vi "Main VI.vi"() -> ()   [LabVIEW 2015]
uses:
  Control 2.ctl
  <vilib>/MakerHub/LINX/Public/Peripherals/Digital/Digital Write 1 Chan.vi
  <vilib>/MakerHub/LINX/Public/Peripherals/Digital/Digital Write N Chans.vi
  <vilib>/MakerHub/LINX/Private/Local IO/LinxDigitalWrite.vi
  <vilib>/MakerHub/LINX/Public/Utilities/Check Channel.vi
  <vilib>/MakerHub/LINX/Public/Utilities/Open Serial.vi
  <vilib>/MakerHub/LINX/Private/Utilties/Generate Error.vi
  <vilib>/MakerHub/LINX/LMH-LINX.lvlib
panel:
  in  "Stop Button":bool caption="Blank Button"
  in  "Blank Button":bool
  out "7":bool
  out "6":bool
  out "5":bool
  out "4":bool
  out "3":bool
  out "2":bool
  in  "Select Pattern":T1(ring)=enum."All Blink"
  out "Error Details":errorcluster
  out "Device Name":string
  in  "Serial Port":refnum<visa-resource-name>="COM4"
  # "ARDUINO LED PATTERN PROGRAM v1.0"
  # "LED Pin Configuration"
  # "Pattern Selection"
  # "Board Settings"
  # "Error Details"
  # "Programmed by Aswin Sarang & Tarun Goyal\nwww.aswinsarang.com\nmail@aswinsarang.com"
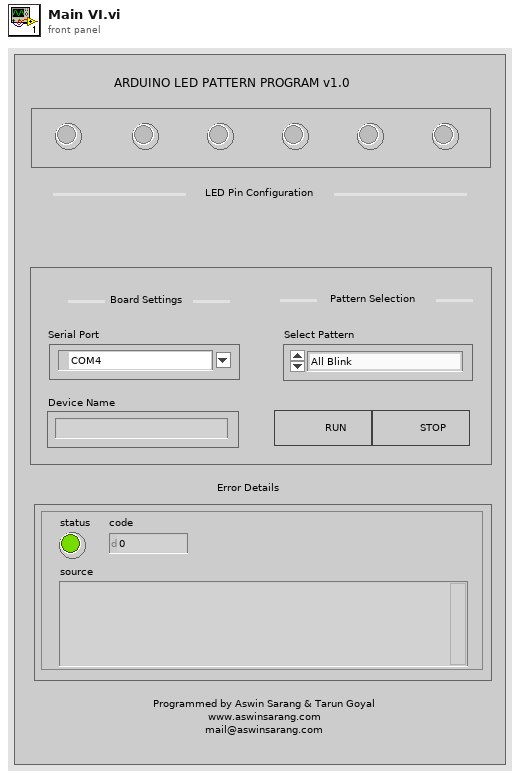
[diagram p1: front panel]
types:
  T1 = enum16{"Open & Close", "Odd & Even", "All Blink", "Running"}
  T2 = typedef "LMH-LINX.lvlib/LINX Ref.ctl" = cluster{"IO":T3, "Interface":T4, "LINX Device Config":T5}
  T3 = typedef "LMH-LINX.lvlib/Platform.ctl" = enum16{"Remote", "Local"}
  T4 = typedef "LMH-LINX.lvlib/Interface.ctl" = enum16{"Serial", "TCP"}
  T5 = typedef "LMH-LINX.lvlib/Device.lvlib/LINX Device Config.ctl" = cluster{"Interface":T4, "COM Port":refnum<visa-resource-name>, "TCP Configuration":T6, "Device Family":u8, "Device ID":u8, "Device Name":string, "TCP Ref":refnum<k5>, "Channels":T7}
  T6 = typedef "LMH-LINX.lvlib/Device.lvlib/TCP Config.ctl" = cluster{"IP Address":string, "Port":u16}
  T7 = typedef "LMH-LINX.lvlib/Channels.ctl" = cluster{"DI":u8[], "DO":u8[], "AI":u8[], "AO":u8[], "PWM":u8[], "QE":u8[], "UART":u8[], "I2C 2":u8[], "SPI":u8[], "CAN":u8[], "Servo":u8[], "AI Ref (V)":dbl, "AI Resolution (Bits)":u8, "AO Ref (V)":dbl, "AO Resolution (Bits)":u8}
  T8 = enum16{"led1", "led2", "led3", "led4", "led5", "led6"}
  T9 = typedef "Control 2.ctl" = u32
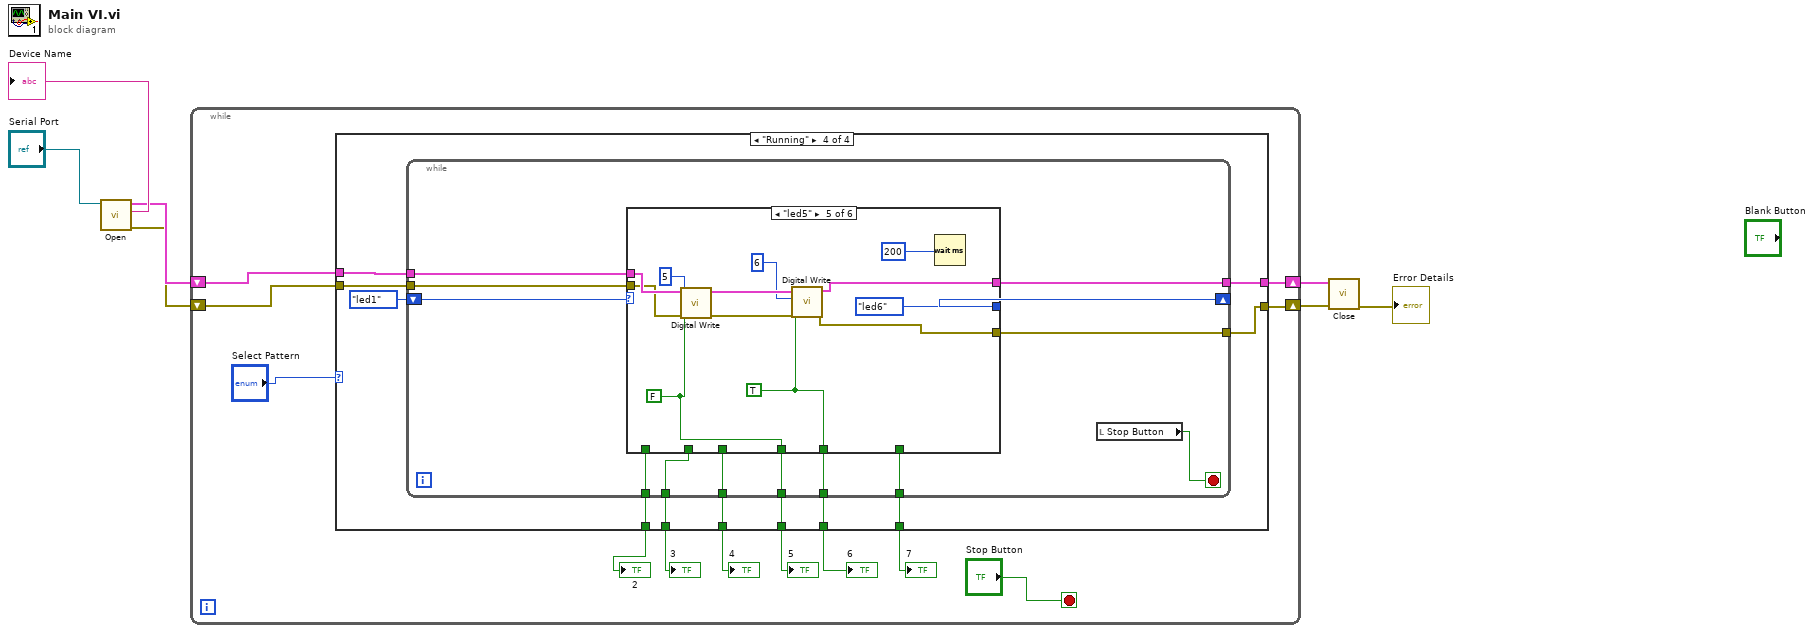
[diagram p0: block diagram]
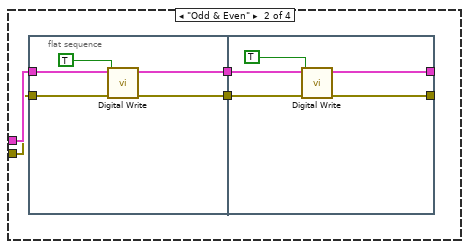
[diagram p3: hidden frame]
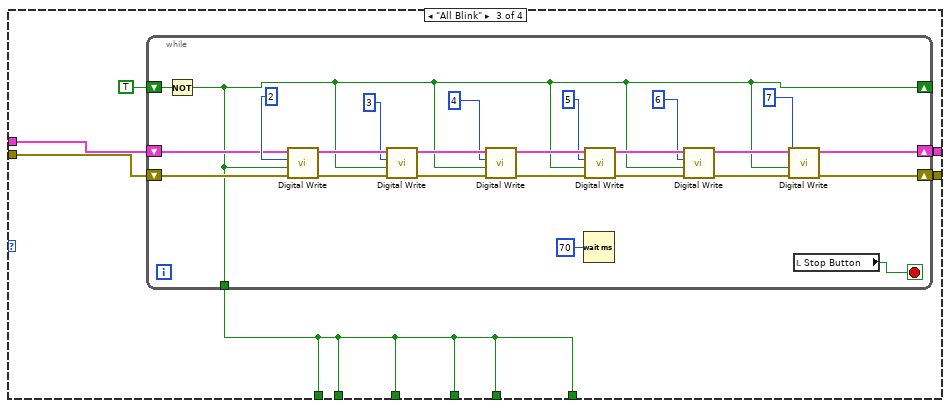
[diagram p4: hidden frame]
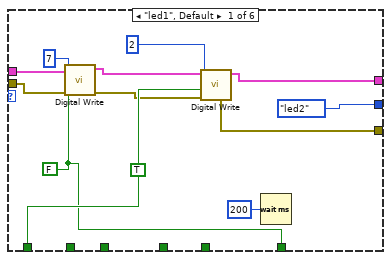
[diagram p5: hidden frame]
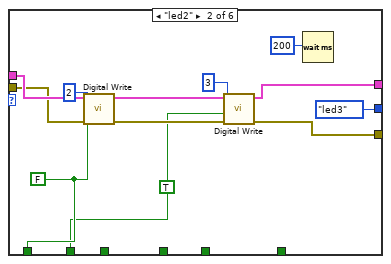
[diagram p6: hidden frame]
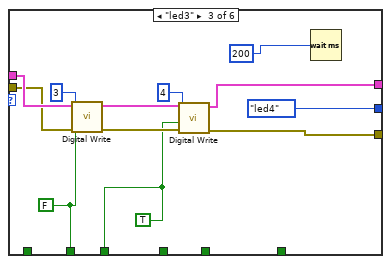
[diagram p7: hidden frame]
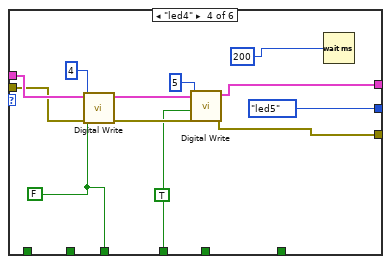
[diagram p8: hidden frame]
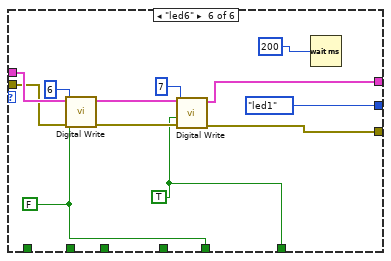
[diagram p9: hidden frame]
diagram:
  n1 = call-poly <vilib>:"Open.vi"("Serial Port"="Serial Port") -> ("Error Out"=w3:errorcluster, "Device Name"=→"Device Name":string, "LINX Resource"=w5:T2)  [unwired: 8 in]
  n2 = while {
    shift-right: [w15] -> w4
    shift-left: w5 -> [w18]
    shift-right: [w14] -> w2
    shift-left: w3 -> [w17]
    stop <- "Stop Button" stop-if-true
    n3 = case shown="\"Running\"" "Select Pattern" {
      tunnel: w18 -> [_ w23 w36 w74]
      tunnel: w17 -> [_ w22 w37 w73]
      tunnel: [_ _ w39 w70] -> w15
      tunnel: [_ _ w38 w69] -> w14
      tunnel: [_ _ w34 w71] -> w13
      tunnel: [_ _ w34 w68] -> w12
      tunnel: [_ _ w34 w67] -> w11
      tunnel: [_ _ w34 w66] -> w10
      tunnel: [_ _ w34 w65] -> w9
      tunnel: [_ _ w34 w64] -> w8
      frame "Open & Close", Default {
      }
      frame "Odd & Even" {
        n4 = flat-sequence {
          tunnel: w23 -> [w28]
          tunnel: [w27] -> w21
          tunnel: w22 -> [w26]
          tunnel: [w25] -> w20
          tunnel: w21 -> [w33]
          tunnel: [w32] -> _
          tunnel: w20 -> [w31]
          tunnel: [w29] -> _
          frame #0 {
            n5 = call-poly <vilib>:"Digital Write.vi"("Error In"=w26, "Output Value"=TRUE, "LINX Resource"=w28) -> ("Error Out"=w25:errorcluster, "LINX Resource"=w27:T2)  [unwired: 7 in]
          }
          frame #1 {
            n6 = call-poly <vilib>:"Digital Write.vi"("Error In"=w31, "Output Value"=TRUE, "LINX Resource"=w33) -> ("Error Out"=w29:errorcluster, "LINX Resource"=w32:T2)  [unwired: 7 in]
          }
        }
      }
      frame "All Blink" {
        n7 = while {
          shift-right: [w52] -> w38
          shift-left: w37 -> [w45]
          shift-right: [w53] -> w39
          shift-left: w36 -> [w44]
          shift-right: [w41] -> _
          shift-left: TRUE -> [w43]
          tunnel: [w41] -> w34
          stop <- w42 stop-if-true
          n8 = Not(x=w43) -> (.not. x?=w41:bool)
          n9 = call-poly <vilib>:"Digital Write.vi"("Error In"=w45, "Output Value"=w41, "DO Channel"=2, "LINX Resource"=w44) -> ("Error Out"=w63:errorcluster, "LINX Resource"=w58:T2)  [unwired: 6 in]
          n10 = call-poly <vilib>:"Digital Write.vi"("Error In"=w63, "Output Value"=w41, "DO Channel"=3, "LINX Resource"=w58) -> ("Error Out"=w62:errorcluster, "LINX Resource"=w57:T2)  [unwired: 6 in]
          n11 = call-poly <vilib>:"Digital Write.vi"("Error In"=w62, "Output Value"=w41, "DO Channel"=4, "LINX Resource"=w57) -> ("Error Out"=w61:errorcluster, "LINX Resource"=w56:T2)  [unwired: 6 in]
          n12 = Wait (ms)(milliseconds to wait=u32 70) -> ()  [unwired: 1 out]
          n13 = call-poly <vilib>:"Digital Write.vi"("Error In"=w61, "Output Value"=w41, "DO Channel"=5, "LINX Resource"=w56) -> ("Error Out"=w60:errorcluster, "LINX Resource"=w55:T2)  [unwired: 6 in]
          n14 = call-poly <vilib>:"Digital Write.vi"("Error In"=w60, "Output Value"=w41, "DO Channel"=6, "LINX Resource"=w55) -> ("Error Out"=w59:errorcluster, "LINX Resource"=w54:T2)  [unwired: 6 in]
          n15 = call-poly <vilib>:"Digital Write.vi"("Error In"=w59, "Output Value"=w41, "DO Channel"=7, "LINX Resource"=w54) -> ("Error Out"=w52:errorcluster, "LINX Resource"=w53:T2)  [unwired: 6 in]
          n16 = local read "Stop Button"() -> (w42:bool)
        }
      }
      frame "Running" {
        n17 = while {
          tunnel: w74 -> [w85]
          tunnel: w73 -> [w84]
          shift-right: [w86] -> _
          shift-left: T8."led1" -> [w87]
          tunnel: [w83] -> w71
          tunnel: [w82] -> w70
          tunnel: [w81] -> w69
          tunnel: [w79] -> w68
          tunnel: [w78] -> w67
          tunnel: [w77] -> w66
          tunnel: [w76] -> w65
          tunnel: [w75] -> w64
          stop <- w80 stop-if-true
          n18 = case shown="\"led5\"" w87 {
            tunnel: [T8."led2" T8."led3" T8."led4" T8."led5" T8."led6" T8."led1"] -> w86
            tunnel: w85 -> [w93 w110 w122 w134 w146 w158]
            tunnel: w84 -> [w91 w109 w117 w129 w143 w153]
            tunnel: [w97 w107 _ _ _ _] -> w83
            tunnel: [w96 w105 w120 w132 w144 w156] -> w82
            tunnel: [w95 w103 w119 w131 w141 w155] -> w81
            tunnel: [_ w101 w114 _ _ _] -> w79
            tunnel: [_ _ w113 w126 _ _] -> w78
            tunnel: [_ _ _ w125 w138 _] -> w77
            tunnel: [_ _ _ _ w137 w150] -> w76
            tunnel: [w90 _ _ _ _ w149] -> w75
            frame "led1", Default {
              w90 = FALSE ("Output Value")
              w97 = TRUE ("Output Value")
              n19 = call-poly <vilib>:"Digital Write.vi"("Error In"=w91, "Output Value"=w90, "DO Channel"=u8 7, "LINX Resource"=w93) -> ("Error Out"=w88:errorcluster, "LINX Resource"=w89:T2)  [unwired: 6 in]
              n20 = call-poly <vilib>:"Digital Write.vi"("Error In"=w88, "Output Value"=w97, "DO Channel"=u8 2, "LINX Resource"=w89) -> ("Error Out"=w95:errorcluster, "LINX Resource"=w96:T2)  [unwired: 6 in]
              n21 = Wait (ms)(milliseconds to wait=T9 200) -> ()  [unwired: 1 out]
            }
            frame "led2" {
              w101 = TRUE ("Output Value")
              w107 = FALSE ("Output Value")
              n22 = call-poly <vilib>:"Digital Write.vi"("Error In"=w109, "Output Value"=w107, "DO Channel"=u8 2, "LINX Resource"=w110) -> ("Error Out"=w104:errorcluster, "LINX Resource"=w106:T2)  [unwired: 6 in]
              n23 = call-poly <vilib>:"Digital Write.vi"("Error In"=w104, "Output Value"=w101, "DO Channel"=u8 3, "LINX Resource"=w106) -> ("Error Out"=w103:errorcluster, "LINX Resource"=w105:T2)  [unwired: 6 in]
              n24 = Wait (ms)(milliseconds to wait=T9 200) -> ()  [unwired: 1 out]
            }
            frame "led3" {
              w113 = TRUE ("Output Value")
              w114 = FALSE ("Output Value")
              n25 = call-poly <vilib>:"Digital Write.vi"("Error In"=w117, "Output Value"=w114, "DO Channel"=u8 3, "LINX Resource"=w122) -> ("Error Out"=w118:errorcluster, "LINX Resource"=w121:T2)  [unwired: 6 in]
              n26 = call-poly <vilib>:"Digital Write.vi"("Error In"=w118, "Output Value"=w113, "DO Channel"=u8 4, "LINX Resource"=w121) -> ("Error Out"=w119:errorcluster, "LINX Resource"=w120:T2)  [unwired: 6 in]
              n27 = Wait (ms)(milliseconds to wait=T9 200) -> ()  [unwired: 1 out]
            }
            frame "led4" {
              w125 = TRUE ("Output Value")
              w126 = FALSE ("Output Value")
              n28 = call-poly <vilib>:"Digital Write.vi"("Error In"=w129, "Output Value"=w126, "DO Channel"=u8 4, "LINX Resource"=w134) -> ("Error Out"=w130:errorcluster, "LINX Resource"=w133:T2)  [unwired: 6 in]
              n29 = call-poly <vilib>:"Digital Write.vi"("Error In"=w130, "Output Value"=w125, "DO Channel"=u8 5, "LINX Resource"=w133) -> ("Error Out"=w131:errorcluster, "LINX Resource"=w132:T2)  [unwired: 6 in]
              n30 = Wait (ms)(milliseconds to wait=T9 200) -> ()  [unwired: 1 out]
            }
            frame "led5" {
              w137 = TRUE ("Output Value")
              w138 = FALSE ("Output Value")
              n31 = call-poly <vilib>:"Digital Write.vi"("Error In"=w143, "Output Value"=w138, "DO Channel"=u8 5, "LINX Resource"=w146) -> ("Error Out"=w142:errorcluster, "LINX Resource"=w145:T2)  [unwired: 6 in]
              n32 = call-poly <vilib>:"Digital Write.vi"("Error In"=w142, "Output Value"=w137, "DO Channel"=u8 6, "LINX Resource"=w145) -> ("Error Out"=w141:errorcluster, "LINX Resource"=w144:T2)  [unwired: 6 in]
              n33 = Wait (ms)(milliseconds to wait=T9 200) -> ()  [unwired: 1 out]
            }
            frame "led6" {
              w149 = TRUE ("Output Value")
              w150 = FALSE ("Output Value")
              n34 = call-poly <vilib>:"Digital Write.vi"("Error In"=w153, "Output Value"=w150, "DO Channel"=u8 6, "LINX Resource"=w158) -> ("Error Out"=w154:errorcluster, "LINX Resource"=w157:T2)  [unwired: 6 in]
              n35 = call-poly <vilib>:"Digital Write.vi"("Error In"=w154, "Output Value"=w149, "DO Channel"=u8 7, "LINX Resource"=w157) -> ("Error Out"=w155:errorcluster, "LINX Resource"=w156:T2)  [unwired: 6 in]
              n36 = Wait (ms)(milliseconds to wait=T9 200) -> ()  [unwired: 1 out]
            }
          }
          n37 = local read "Stop Button"() -> (w80:bool)
        }
      }
    }
    "2" <- w13
    "3" <- w12
    "4" <- w11
    "5" <- w10
    "6" <- w9
    "7" <- w8
  }
  n38 = call <vilib>:"Close.vi"("Error In"=w2, "LINX Resource"=w4) -> ("Error Out"=→"Error Details":errorcluster)  [unwired: 9 in]
